vi "buildmScript.vi"(8 "error in (no error)":errorcluster, 9 "Jpeg path":path, 10 "Sudoku array":string[][](array[string]), 11 "Current path":path) -> (0 "error out":errorcluster)   [LabVIEW 2020]
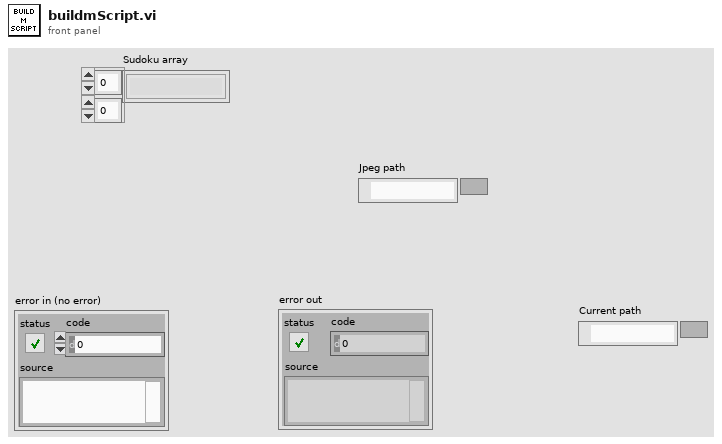
[diagram p1: front panel]
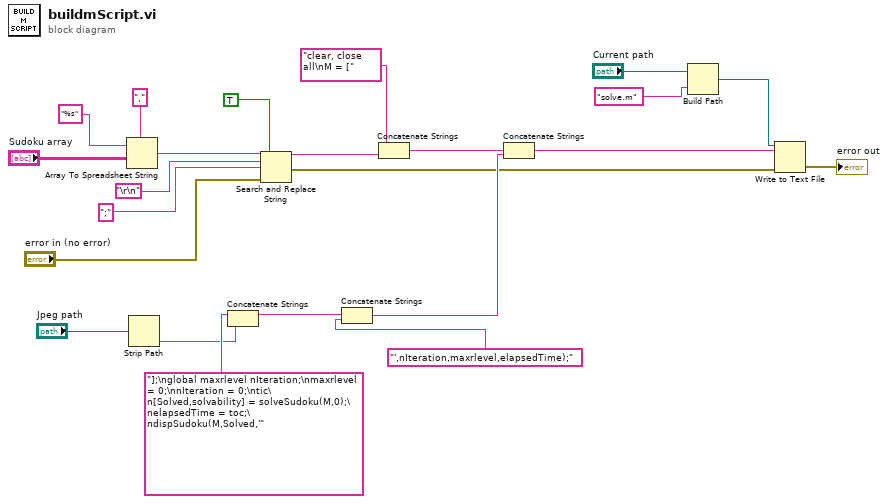
[diagram p0: block diagram]
diagram:
  n1 = Array To Spreadsheet String(delimiter (Tab)=",", array="Sudoku array", 3:"%s") -> (spreadsheet string=w20:string)
  n2 = Strip Path(path="Jpeg path") -> (name=w10:string)  [unwired: 1 out]
  n3 = Concatenate Strings("];\nglobal maxrlevel nIteration;\nmaxrlevel = 0;\nnIteration = 0;\ntic\n[Solved,solvability] = solveSudoku(M,0);\nelapsedTime = toc;\ndispSudoku(M,Solved,'", w10) -> (w9:string)
  n4 = Search and Replace String(replace all?=TRUE, input string=w20, search string="\r\n", replace string=";", error in="error in (no error)") -> (result string=w15:string, error out=w2:errorcluster)  [unwired: 3 in, 2 out]
  n5 = Concatenate Strings(w9, "',nIteration,maxrlevel,elapsedTime);") -> (w7:string)
  n6 = Concatenate Strings("clear, close all\nM = [", w15) -> (w13:string)
  n7 = Concatenate Strings(w13, w7) -> (w3:string)
  n8 = Build Path(base path="Current path", name or relative path="solve.m") -> (appended path=w4:path)
  n9 = Write to Text File(file (use dialog)=w4, text=w3, error in=w2) -> (error out=→"error out":errorcluster)  [unwired: 1 in, 2 out]
